vi "Set Debug Data Listener.vi"(8 "error in (no error)":errorcluster, 10 "Broadcast Reg":refnum<event-registration>, 11 "Broadcast Message Receiver In":refnum<class "Broadcast Message Receiver.lvclass">) -> (0 "error out":errorcluster, 3 "Broadcast Message Receiver Out":refnum<class "Broadcast Message Receiver.lvclass">)   [LabVIEW 2020, in "Broadcast Message Receiver.lvclass"]
uses:
  Broadcast Message Receiver.lvclass
  Broadcast Message Receiver.lvclass/Broadcast Message Receiver.ctl
  C:/Users/anton/Documents/GitHub/triarc-debugger/source/Process/Debug Process.lvclass
  C:/Users/anton/Documents/GitHub/triarc-debugger/source/Broadcast Message Receiver/Broadcast Message Receiver.lvclass
  Process/Debug Process.lvclass
  <vilib>/Astemes/Triarc Framework/Process/Protected/Broadcasting/Broadcast Message Cluster.ctl
  <vilib>/Astemes/Triarc Framework/Process/Process.lvclass
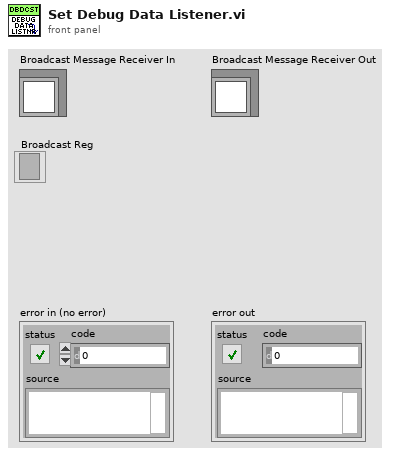
[diagram p1: front panel]
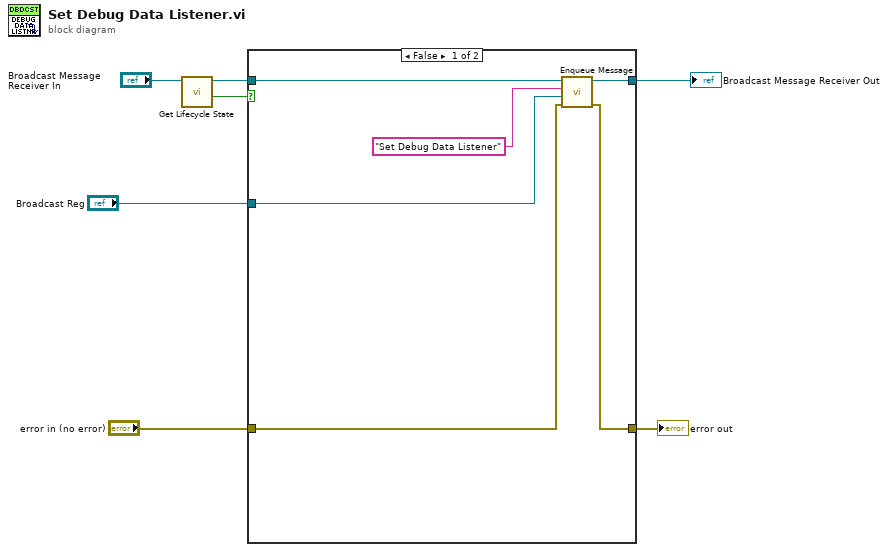
[diagram p0: block diagram]
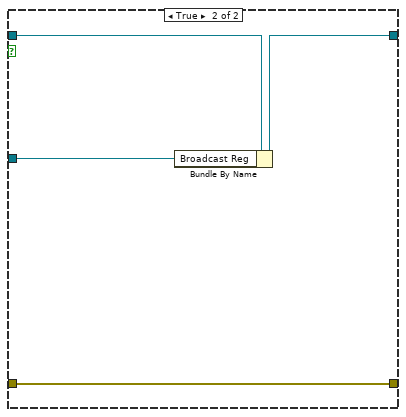
[diagram p2: hidden frame]
diagram:
  n1 = call "Get Lifecycle State.vi"("Process In"="Broadcast Message Receiver In") -> ("In Process Loop?"=w3:bool, "Process Out"=w6:refnum<class "Broadcast Message Receiver.lvclass">)  [unwired: 7 in, 2 out]
  n2 = case shown="False" w3 {
    tunnel: w6 -> [w13 w17]
    tunnel: [w12 w15] -> w5
    tunnel: "error in (no error)" -> [w8 w16]
    tunnel: [w9 w16] -> w4
    tunnel: "Broadcast Reg" -> [w11 w14]
    frame False {
      n3 = call "Enqueue Message.vi"("error in (no error)"=w8, "Message Data"=w11, "Message"="Set Debug Data Listener" ("API Message"), "Process In"=w13) -> ("error out"=w9:errorcluster, "Process Out"=w12:refnum<class "Broadcast Message Receiver.lvclass">)  [unwired: 6 in]
    }
    frame True {
      n4 = Bundle By Name(cluster=w17, "Broadcast Reg"=w14) -> (w15:refnum<class "Broadcast Message Receiver.lvclass">)
    }
  }
  "error out" <- w4
  "Broadcast Message Receiver Out" <- w5
